vi "Init Single.vi"(10 "value":T1) -> (3 "Msg out":refnum<class "Msg.lvclass">)   [LabVIEW 2023, in "CmdAnalogMultiple.lvlib" / "Msg.lvclass"]
uses:
  Msg.lvclass
  Msg.lvclass/Msg.ctl
  CmdAnalog/Data.ctl
  CmdAnalog/CmdAnalog.lvlib
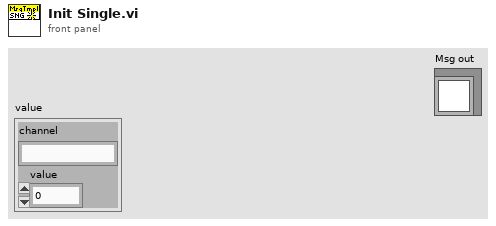
[diagram p1: front panel]
types:
  T1 = typedef "CmdAnalog.lvlib/Data.ctl" = cluster{"channel":string, "value":dbl}
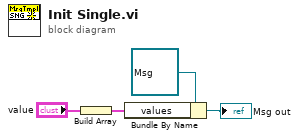
[diagram p0: block diagram]
diagram:
  n1 = Build Array("value") -> (w1:T1[])
  n2 = Bundle By Name(cluster=refnum<class "Msg.lvclass"> refnum ("Msg out"), "values"=w1) -> (→"Msg out":refnum<class "Msg.lvclass">)
